vi "Write Qsp.vi"(8 "error in (no error)":errorcluster, 10 "Qsp":sgl, 11 "VC Data in":refnum<class "VC Data.lvclass">) -> (0 "error out":errorcluster, 3 "VC Data out":refnum<class "VC Data.lvclass">)   [LabVIEW 2015, in "VC Data.lvclass"]
uses:
  VC Data.lvclass
  VC Data.lvclass/VC Data.ctl
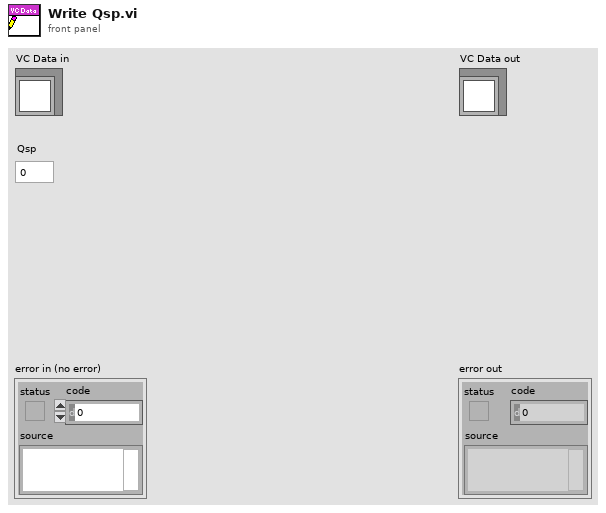
[diagram p1: front panel]
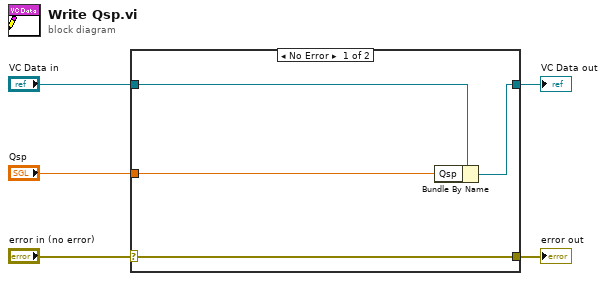
[diagram p0: block diagram]
diagram:
  n1 = case shown="No Error" "error in (no error)" {
    selector: "error in (no error)" -> [w9 w10]
    tunnel: [w9 w10] -> w4
    tunnel: [w7 w11] -> w2
    tunnel: "VC Data in" -> [w8 w11]
    tunnel: "Qsp" -> [w6 _]
    frame No Error {
      n2 = Bundle By Name(cluster=w8, "Qsp"=w6) -> (w7:refnum<class "VC Data.lvclass">)
    }
    frame Error {
    }
  }
  "error out" <- w4
  "VC Data out" <- w2
